vi "Target 2 Command Data.vi"(10 "Current \nPosition":dbl[](array[numeric]), 11 "Command Data":T1={"Displacements"=[4.0, 3.0, 0.0, 0.0, 0.0, 0.0], "Command Type"=[enum."<None>", enum."Displacement", enum."<None>", enum."Force", enum."<None>", enum."Force"], "Forces"=[0.0, 0.0, 0.0, 6.0, 0.0, 8.0]}) -> (2 "Output":dbl[](array[numeric]))   [LabVIEW 2009]
uses:
  Target Data.ctl
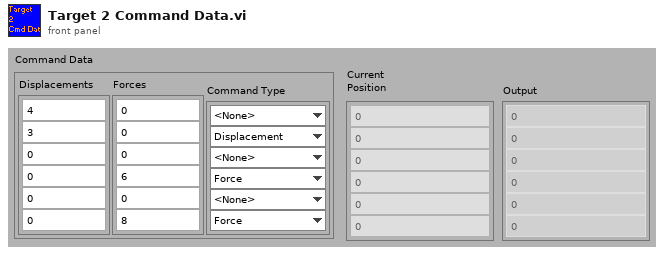
[diagram p1: front panel]
types:
  T1 = typedef "Target Data.ctl" = cluster{"Displacements":dbl[], "Command Type":enum16{"<None>", "Displacement", "Force"}[], "Forces":dbl[]}
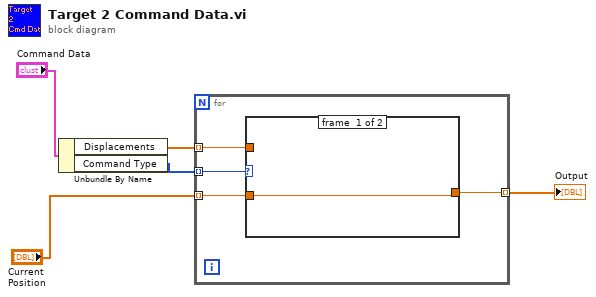
[diagram p0: block diagram]
diagram:
  n1 = Unbundle By Name("Command Data") -> ("Displacements"=w3:dbl[], "Command Type"=w4:enum16{"<None>", "Displacement", "Force"}[])
  n2 = for {
    tunnel: w4 -> [w9] mode=indexing
    tunnel: w3 -> [w8] mode=indexing
    tunnel: "Current \nPosition" -> [w7] mode=indexing
    tunnel: [w6] -> w1 mode=indexing
    n3 = case shown="\"<None>\", Default" w9 {
      tunnel: w8 -> [_ w11]
      tunnel: w7 -> [w10 _]
      tunnel: [w10 w11] -> w6
      frame #0 {
      }
      frame #1 {
      }
    }
  }
  "Output" <- w1
